vi "Func_ConvertColors.vi"(8 "error in (no error)":errorcluster, 9 "Color Box":u32(colorbox), 10 "New Type":string, 11 "Path":path) -> (0 "error out":errorcluster)   [LabVIEW 2010, in "TemplateGenerator.lvlib"]
uses:
  TemplateGenerator.lvlib
  <vilib>/LabVIEW Icon API/LabVIEW Icon API.lvlib
  <vilib>/picture/picture.llb/imagedata.ctl
  <vilib>/Utility/miscctls.llb/LVPoint32TypeDef.ctl
  <vilib>/LabVIEW Icon API/API_User Layer Data.ctl
  <vilib>/LabVIEW Icon API/lv_icon/Controls/Layer.ctl
  <vilib>/LabVIEW Icon API/lv_icon/Classes/Layer/Layer.lvclass
  <vilib>/LabVIEW Icon API/lv_icon/Classes/Icon/Icon.lvclass
  <vilib>/LabVIEW Icon API/lv_icon/Controls/LayerType.ctl
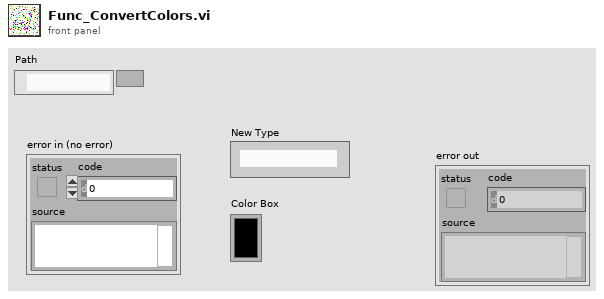
[diagram p1: front panel]
types:
  T1 = typedef "LayerType.ctl" = enum16{"Graphic", "Text", "Tool", "Graphic Drop"}
  T2 = typedef "Layer.ctl" = cluster{"LayerIcon":picture, "LayerName":string, "Opacity":u8, "Visibility?":bool}
  T3 = typedef "LabVIEW Icon API.lvlib/API_User Layer Data.ctl" = cluster{"Layer name":string, "Origin":T4, "Icon image data":T5}
  T4 = typedef "LVPoint32TypeDef.ctl" = cluster{"Horizontal":i32, "Vertical":i32}
  T5 = typedef "imagedata.ctl" = cluster{"image type":i32, "image depth":i32, "image":u8[], "mask":u8[], "colors":u32[], "Rectangle":cluster{"left":i16, "top":i16, "right":i16, "bottom":i16}}
  T6 = cluster{"horizontal":enum16{"left", "center", "right"}, "vertical":enum16{"top", "center", "bottom"}}
  T7 = cluster{"Font Name:":string, "Size":i16, "Strikeout?":bool, "Italic?":bool, "Underline?":bool, "Outline?":bool, "Shadow?":bool, "Bold?":bool}
  T8 = enum16{"User-specified Font", "Application Font", "System Font", "Dialog Font"}
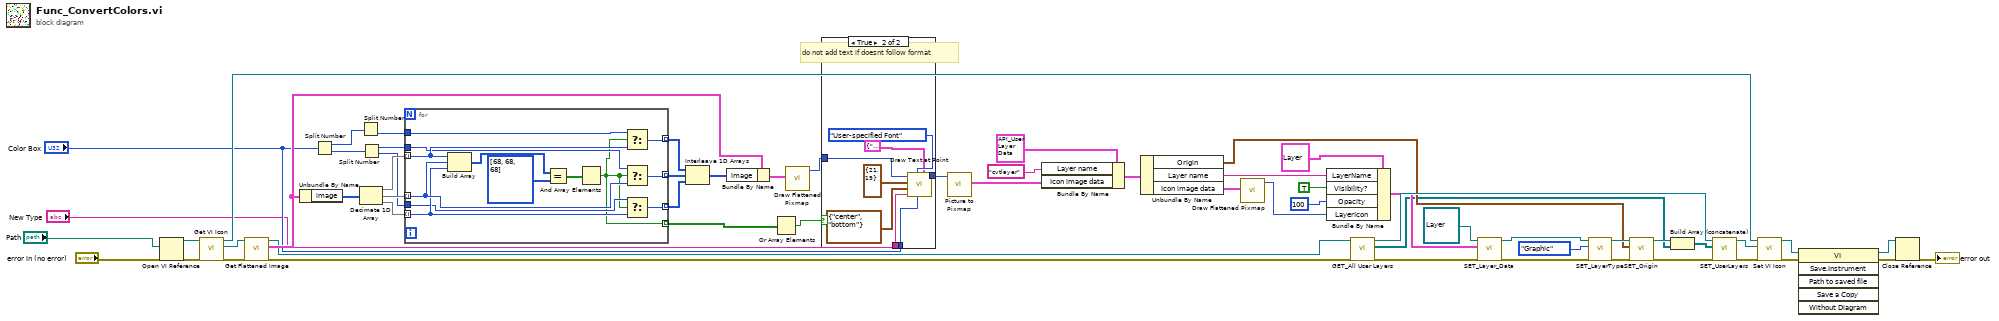
[diagram p0: block diagram]
diagram:
  n1 = Open VI Reference(vi path="Path", error in (no error)="error in (no error)") -> (vi reference=w6:refnum<vi>, error out=w5:errorcluster)  [unwired: 4 in]
  n2 = call <vilib>:"Get VI Icon.vi"("error in (no error)"=w5, "VI Refnum in"=w6) -> ("error out"=w60:errorcluster, "Icon"=w61:refnum<class "Icon.lvclass">, "VI Refnum out"=w18:refnum<vi>)  [unwired: 7 in]
  n3 = call <vilib>:"Get Flattened Image.vi"("error in (no error)"=w60, "lv_icon.lvlib:Icon.lvclass in"=w61) -> ("error out"=w19:errorcluster, "Color Image"=w47:T5, "lv_icon.lvlib:Icon.lvclass out"=w20:refnum<class "Icon.lvclass">)  [unwired: 6 in, 1 out]
  n4 = Unbundle By Name(w47) -> ("image"=w57:u8[])
  n5 = Split Number(x="Color Box") -> (hi(x)=w58:u16, lo(x)=w59:u16)
  n6 = Split Number(x=w58) -> (lo(x)=w50:u8)  [unwired: 1 out]
  n7 = Decimate 1D Array(w57) -> (w56:u8[], w55:u8[], w54:u8[])
  n8 = Split Number(x=w59) -> (hi(x)=w49:u8, lo(x)=w48:u8)
  n9 = for {
    tunnel: w56 -> [w71] mode=indexing
    tunnel: w55 -> [w70] mode=indexing
    tunnel: w54 -> [w69] mode=indexing
    tunnel: [w68] -> w53 mode=indexing
    tunnel: [w67] -> w52 mode=indexing
    tunnel: [w66] -> w51 mode=indexing
    tunnel: w50 -> [w65]
    tunnel: w49 -> [w64]
    tunnel: w48 -> [w63]
    tunnel: [w62] -> w2 mode=indexing
    n10 = Build Array(w71, w70, w69) -> (w74:u8[])
    n11 = Equal?(x=w74, y=u8[] [68, 68, 68]) -> (x = y?=w72:bool[])
    n12 = And Array Elements(Boolean array=w72) -> (logical AND=w62:bool)
    n13 = Select(t=w65, s=w62, f=w71) -> (s? t:f=w66:u8)
    n14 = Select(t=w64, s=w62, f=w70) -> (s? t:f=w67:u8)
    n15 = Select(t=w63, s=w62, f=w69) -> (s? t:f=w68:u8)
  }
  n16 = Interleave 1D Arrays(w51, w52, w53) -> (w46:u8[])
  n17 = Bundle By Name(cluster=w47, "image"=w46) -> (w45:T5)
  n18 = Or Array Elements(Boolean array=w2) -> (logical OR=w1:bool)
  n19 = call <vilib>:"Draw Flattened Pixmap.vi"("image data"=w45) -> ("new picture"=w21:picture)  [unwired: 8 in]
  n20 = case shown="True" w1 {
    tunnel: [w75 w83] -> w22
    tunnel: w21 -> [w75 w81]
    tunnel: "Color Box" -> [_ w77]
    tunnel: "New Type" -> [_ w76]
    frame False {
    }
    frame True {
      # "do not add text if doesnt follow format"
      n21 = call <vilib>:"Draw Text at Point.vi"("[user-specified font]"=T7 {"Font Name:"="Small Fonts", "Size"=9, "Strikeout?"=FALSE, "Italic?"=FALSE, "Underline?"=FALSE, "Outline?"=FALSE, "Shadow?"=FALSE, "Bold?"=FALSE}, "text color(black)"=w77, "desired font(Application)"=T8."User-specified Font", "text"=w76, "alignment(left, top)"=T6 {"horizontal"=enum."center", "vertical"=enum."bottom"}, "origin"=cluster{"x":i16, "y":i16} {"x"=21, "y"=19}, "picture"=w81) -> ("new picture"=w83:picture)  [unwired: 3 in, 1 out]
    }
  }
  n22 = call <vilib>:"Picture to Pixmap.vi"("picture"=w22) -> ("image data"=w43:T5)  [unwired: 9 in, 1 out]
  n23 = Bundle By Name(cluster=T3 {"Layer name"="", "Origin"={"Horizontal"=0, "Vertical"=0}, "Icon image data"={"image type"=0, "image depth"=0, "image"=[], "mask"=[], "colors"=[], "Rectangle"={"left"=0, "top"=0, "right"=0, "bottom"=0}}} ("User layer"), "Layer name"="cvtlayer", "Icon image data"=w43) -> (w23:T3)
  n24 = Unbundle By Name(w23) -> ("Origin"=w27:T4, "Layer name"=w29:string, "Icon image data"=w25:T5)
  n25 = call <vilib>:"Draw Flattened Pixmap.vi"("image data"=w25) -> ("new picture"=w24:picture)  [unwired: 8 in]
  n26 = Bundle By Name(cluster=T2 {"LayerIcon"=bytes[0], "LayerName"="", "Opacity"=0, "Visibility?"=FALSE} ("Data"), "LayerName"=w29, "Visibility?"=TRUE, "Opacity"=u8 100, "LayerIcon"=w24) -> (w32:T2)
  n27 = call-dynamic "GET_All User Layers.vi"("error in (no error)"=w19, "Icon.lvclass in"=w20) -> ("error out"=w37:errorcluster, "User Layer"=w14:refnum<class "Layer.lvclass">[], "Icon.lvclass out"=w38:refnum<class "Icon.lvclass">)  [unwired: 7 in]
  n28 = call-dynamic "SET_Layer_Data.vi"("error in (no error)"=w37, "Data"=w32, "Layer.lvclass in"=refnum<class "Layer.lvclass"> refnum) -> ("error out"=w33:errorcluster, "Layer.lvclass out"=w31:refnum<class "Layer.lvclass">)  [unwired: 1 in, 6 out]
  n29 = call-dynamic "SET_LayerType.vi"("error in (no error)"=w33, "Type"=LayerType."Graphic", "Layer.lvclass in"=w31) -> ("error out"=w26:errorcluster, "Layer.lvclass out"=w28:refnum<class "Layer.lvclass">)  [unwired: 7 out]
  n30 = call-dynamic "SET_Origin.vi"("error in (no error)"=w26, "Point32"=w27, "Layer.lvclass in"=w28) -> ("error out"=w36:errorcluster, "Layer.lvclass out"=w15:refnum<class "Layer.lvclass">)  [unwired: 7 in]
  n31 = Build Array (concatenate)(w15, w14) -> (w39:refnum<class "Layer.lvclass">[])
  n32 = call-dynamic "SET_UserLayers.vi"("error in (no error)"=w36, "Layers"=w39, "Icon.lvclass in"=w38) -> ("error out"=w16:errorcluster, "Icon.lvclass out"=w17:refnum<class "Icon.lvclass">)  [unwired: 7 in]
  n33 = call <vilib>:"Set VI Icon.vi"("error in (no error)"=w16, "Icon"=w17, "VI Refnum in"=w18) -> ("error out"=w9:errorcluster, "VI Refnum out"=w10:refnum<vi>)  [unwired: 7 in]
  n34 = invoke class="VI" method="Save.Instrument"(reference=w10, error in=w9) -> (reference out=w8:refnum<vi>, error out=w11:errorcluster)  [unwired: 4 in, 4 out]
  n35 = Close Reference(reference=w8, error in (no error)=w11) -> (error out=→"error out":errorcluster)
